vi "Write Cooler ON_OFF.vi"(8 "error in (no error)":errorcluster, 10 "Cooler ON/OFF":u8, 11 "Cooler in":refnum<class "Simulated_Cooler.lvclass">) -> (0 "error out":errorcluster, 3 "Cooler out":refnum<class "Simulated_Cooler.lvclass">)   [LabVIEW 2018, in "Simulated_Cooler.lvclass"]
uses:
  Simulated_Cooler.lvclass
  Simulated_Cooler.lvclass/Simulated_Cooler.ctl
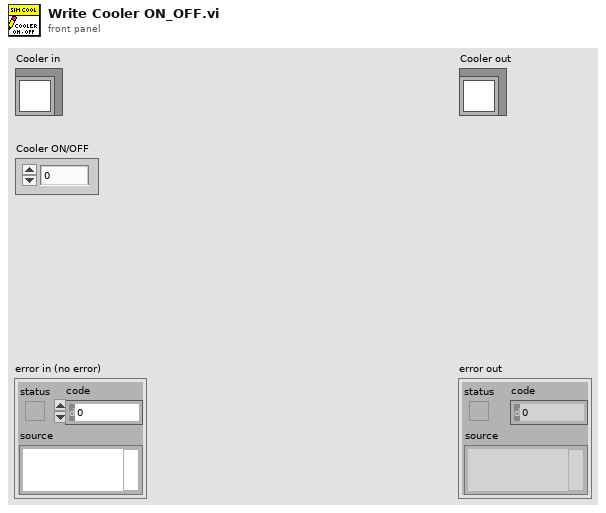
[diagram p1: front panel]
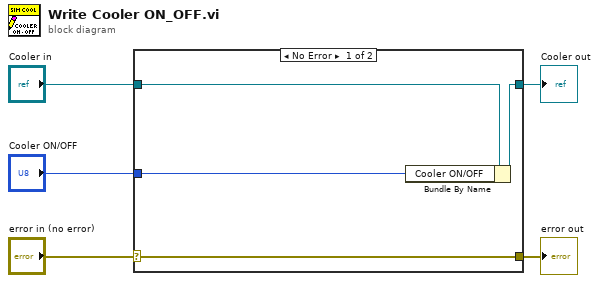
[diagram p0: block diagram]
diagram:
  n1 = case shown="No Error" "error in (no error)" {
    selector: "error in (no error)" -> [w9 w10]
    tunnel: [w9 w10] -> w4
    tunnel: [w7 w11] -> w2
    tunnel: "Cooler in" -> [w8 w11]
    tunnel: "Cooler ON/OFF" -> [w6 _]
    frame No Error {
      n2 = Bundle By Name(cluster=w8, "Cooler ON/OFF"=w6) -> (w7:refnum<class "Simulated_Cooler.lvclass">)
    }
    frame Error {
    }
  }
  "error out" <- w4
  "Cooler out" <- w2
